vi "LibXML_GetAttrName.vi"(8 "error in":errorcluster, 10 "attribute":u32) -> (0 "error out":errorcluster, 3 "lvstring":string)   [LabVIEW 2019, in "Tools.lvlib" / "LibXML.lvlib"]
doc: "Get the name of attrib at attrib pointer (U32) inut."
uses:
  LibXML.lvlib
  Error Cluster From Error Code_subroutine.vi
  <vilib>/Utility/error.llb/Trim Whitespace.vi
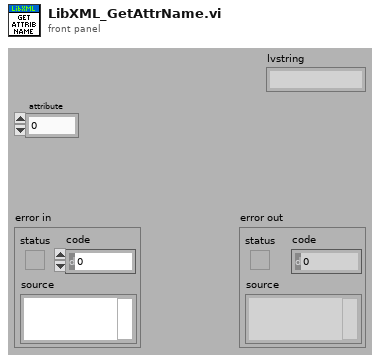
[diagram p1: front panel]
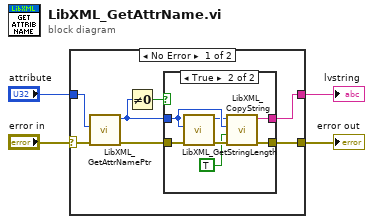
[diagram p0: block diagram]
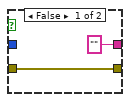
[diagram p2: hidden frame]
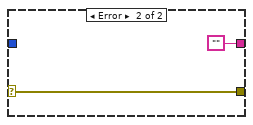
[diagram p3: hidden frame]
diagram:
  n1 = case shown="No Error" "error in" {
    selector: "error in" -> [w10 w22]
    tunnel: [w9 w22] -> w3
    tunnel: [w6 ""] -> w2
    tunnel: "attribute" -> [w5 _]
    frame No Error {
      n2 = call "LibXML_GetAttrNamePtr.vi"("error in"=w10, "attribute"=w5) -> ("error out"=w11:errorcluster, "attribute name ptr  out"=w8:u32)  [unwired: 8 in]
      n3 = Not Equal To 0?(x=w8) -> (x != 0?=w7:bool)
      n4 = case shown="True" w7 {
        tunnel: ["" ("lvstring") w20] -> w6
        tunnel: w11 -> [w13 w19]
        tunnel: w8 -> [_ w17]
        tunnel: [w13 w15] -> w9
        frame False {
        }
        frame True {
          n5 = call "LibXML_GetStringLength.vi"("error in"=w19, "string pointer"=w17) -> ("error out"=w18:errorcluster, "string length"=w16:i32)  [unwired: 4 in]
          n6 = call "LibXML_CopyString.vi"("error in"=w18, "free pointer?"=TRUE, "string pointer"=w17, "length"=w16) -> ("error out"=w15:errorcluster, "lvstring"=w20:string)  [unwired: 6 in]
        }
      }
    }
    frame Error {
    }
  }
  "error out" <- w3
  "lvstring" <- w2
